vi "1002213 pca test support.vi"() -> ()   [LabVIEW 2013]
panel:
  in  "USB Serial Port":refnum<visa-resource-name>
  in  "Quectel USB AT port":refnum<visa-resource-name>
  out "error out":errorcluster
  in  "error in (no error)":errorcluster
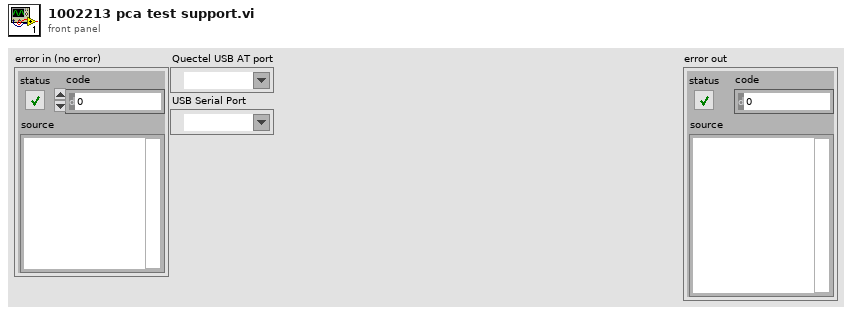
[diagram p1: front panel]
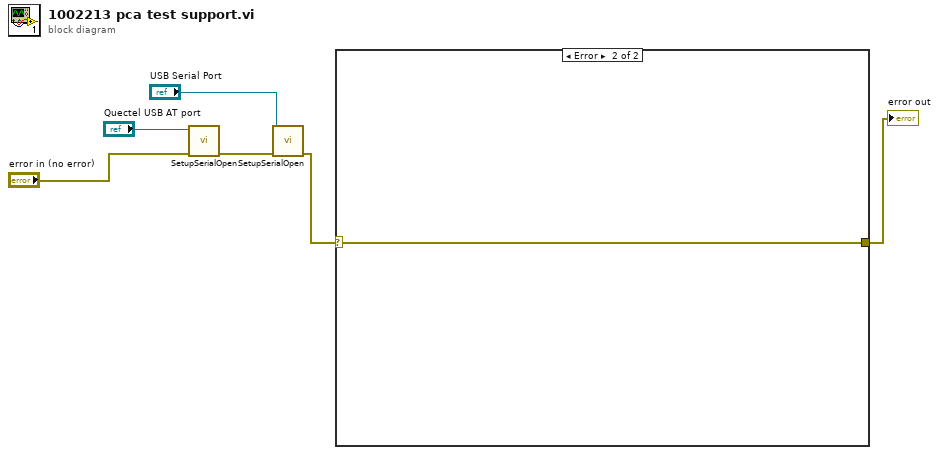
[diagram p0: block diagram]
diagram:
  n1 = call "SetupSerialOpen.vi"("error in (no error)"="error in (no error)", "VISA Refnum in"="Quectel USB AT port") -> ("error out"=w4:errorcluster)  [unwired: 8 in, 1 out]
  n2 = call "SetupSerialOpen.vi"("error in (no error)"=w4, "VISA Refnum in"="USB Serial Port") -> ("error out"=w2:errorcluster)  [unwired: 8 in, 1 out]
  n3 = case shown="Error" w2 {
    selector: w2 -> [w7 w8]
    tunnel: [w7 w8] -> w1
    frame No Error {
    }
    frame Error {
    }
  }
  "error out" <- w1
